vi "S4GUI.vi"(7 "Tab ObsEng":enum32{"Obs", "CCD modes", "Eng"}(tab)) -> ()   [LabVIEW 2018] (continued)
            n1128 = Equal?(x=w198, y=w197) -> (x = y?=w194:bool)
            n1129 = Or(x=w195, y=w194) -> (x .or. y?=w193:bool)
            n1130 = property on="Last Error" class="Str"(error in=w216, "Blinking"=w193) -> (error out=w199:errorcluster)  [unwired: 1 in, 1 out]
            n1131 = call "Read Instrument.lvclass.vi"("error in (no error)"=w199, "S4ACS_GUI in"=w201) -> ("error out"=w205:errorcluster, "Instrument.lvclass"=w204:refnum<class "Instrument.lvclass">, "S4ACS_GUI out"=w203:refnum<class "S4GUI.lvclass">)  [unwired: 7 in]
            n1132 = call-dynamic "Read mode.vi"("error in (no error)"=w205, "Instrument in"=w204) -> ("error out"=w202:errorcluster, "mode"=w206:bool)  [unwired: 7 in, 1 out]
            n1133 = while {
              tunnel: w206 -> [w249]
              shift-right: [w245] -> _
              shift-left: _ -> [w248]
              shift-right: [w246] -> _
              shift-left: _ -> [w247]
              stop <- TRUE stop-if-true
              n1134 = case shown="False" w249 {
                tunnel: w248 -> [w251 w270]
                tunnel: [w252 w269] -> w245
                tunnel: w247 -> [w254 w268]
                tunnel: [w253 w267] -> w246
                frame True {
                  # "polarimetria"
                  n1135 = case shown="False" w254 {
                    selector: w254 -> [w264 w266]
                    tunnel: [w263 w266] -> w253
                    tunnel: [FALSE FALSE] -> w252
                    tunnel: w251 -> [_ _]
                    frame False {
                      w261 = 11
                      w258 = 80
                      w257 = 12900
                      # "Valor médio\ndo curso do foco."
                      n1136 = local write "Start focus"(w257) -> ()
                      n1137 = local write "Step focus"(w258) -> ()
                      n1138 = local write "#steps"(w261) -> ()
                      n1139 = Quotient & Remainder(x=w261, y=2) -> (floor(x/y)=w259:i32)  [unwired: 1 out]
                      n1140 = Multiply(x=w258, y=w259) -> (x*y=w256:i32)
                      n1141 = Add(x=w257, y=w256) -> (x+y=w255:i32)
                      n1142 = local write "Target focus 2"(w255) -> ()
                      n1143 = local write "Target focus"(w255) -> ()
                      n1144 = Not(x=w264) -> (.not. x?=w263:bool)
                    }
                    frame True {
                    }
                  }
                }
                frame False {
                  # "fotometria"
                  n1145 = case shown="False" w270 {
                    selector: w270 -> [w279 w282]
                    tunnel: [w278 w282] -> w269
                    tunnel: w268 -> [_ _]
                    tunnel: [FALSE FALSE] -> w267
                    frame False {
                      w274 = 11
                      w273 = 100
                      w272 = 13400
                      # "Valor médio\ndo curso do foco."
                      n1146 = local write "Start focus"(w272) -> ()
                      n1147 = local write "Step focus"(w273) -> ()
                      n1148 = local write "#steps"(w274) -> ()
                      n1149 = Quotient & Remainder(x=w274, y=2) -> (floor(x/y)=w276:i32)  [unwired: 1 out]
                      n1150 = Multiply(x=w273, y=w276) -> (x*y=w275:i32)
                      n1151 = Add(x=w272, y=w275) -> (x+y=w271:i32)
                      n1152 = local write "Target focus"(w271) -> ()
                      n1153 = local write "Target focus 2"(w271) -> ()
                      n1154 = Not(x=w279) -> (.not. x?=w278:bool)
                    }
                    frame True {
                    }
                  }
                }
              }
            }
          }
        }
        n1155 = call-dynamic "Read exit.vi"("error in (no error)"=w141, "S4GUI in"=w142) -> ("error out"=w139:errorcluster, "exit"=w138:bool, "S4GUI out"=w140:refnum<class "S4GUI.lvclass">)  [unwired: 7 in]
      }
      event "Set CCD mode": Value Change {
        w1932 = i16 1 items=["Cooler OFF", "Cooler ON"] ("Cooler ON/OFF")
        w1946 = i16 1 items=["Cooler OFF", "Cooler ON"] ("Cooler ON/OFF")
        w1962 = i16 1 items=["Cooler OFF", "Cooler ON"] ("Cooler ON/OFF")
        w1982 = i16 1 items=["Cooler OFF", "Cooler ON"] ("Cooler ON/OFF")
        # "Sinaliza que houve requisição de SET CCD mode"
        n1156 = event-data() -> ()  [unwired: 1 in, 6 out]
        n1157 = call-dynamic "Write User Event.vi"("error in (no error)"=w2140, "User Event"="SET CCD mode ", "S4GUI in"=w2139) -> ("error out"=w1927:errorcluster, "S4GUI out"=w1926:refnum<class "S4GUI.lvclass">)  [unwired: 7 in]
        n1158 = call-dynamic "Write SET request.vi"("error in (no error)"=w1927, "SET request"=TRUE, "S4GUI in"=w1926) -> ("error out"=w1924:errorcluster, "S4GUI out"=w1925:refnum<class "S4GUI.lvclass">)  [unwired: 7 in]
        n1159 = call-dynamic "Read CCD mode.vi"("error in (no error)"=w1924, "S4GUI in"=w1925) -> ("error out"=w2137:errorcluster, "CCD mode"=w2138:T29, "S4GUI out"=w2136:refnum<class "S4GUI.lvclass">)  [unwired: 7 in]
        n1160 = Bundle By Name(cluster=w2138, "FTM"="FTM", "AQM"="AQM", "SZM"="SZM", "EM gain"="EM Gain") -> (w2135:T29)
        n1161 = call-dynamic "Write CCD mode.vi"("error in (no error)"=w2137, "CCD mode"=w2135, "S4GUI in"=w2136) -> ("error out"=w1993:errorcluster, "S4GUI out"=w1994:refnum<class "S4GUI.lvclass">)  [unwired: 7 in]
        n1162 = call-dynamic "LoadCCDmode.vi"("error in (no error)"=w1993, "S4GUI in"=w1994) -> ("error out"=w1992:errorcluster, "S4GUI out"=w1991:refnum<class "S4GUI.lvclass">)  [unwired: 8 in]
        n1163 = call-dynamic "Read Parameters CCD modes.vi"("error in (no error)"=w1992, "S4GUI in"=w1991) -> ("error out"=w1990:errorcluster, "Parameters CCD modes"=w1995:T5, "S4GUI out"=w1989:refnum<class "S4GUI.lvclass">)  [unwired: 7 in]
        n1164 = Unbundle By Name(w1995) -> ("CCD \nEM Mode"=w2127:u8, "Readout\nRate"=w1987:u8)
        n1165 = case shown="0, Default" w2127 {
          tunnel: [string[] ["30 MHz", "20 MHz", "10 MHz", "1 MHz"] ("Strings []") string[] ["1 MHz", "0.1 MHz"] ("Strings []")] -> w2128
          frame 0, Default {
          }
          frame 1 {
          }
        }
        n1166 = flat-sequence {
          tunnel: w2128 -> [w2274]
          tunnel: w2127 -> [w2275]
          tunnel: [w2275] -> w2129
          tunnel: w1995 -> [w2281]
          tunnel: [w2280] -> w1988
          tunnel: w2129 -> [w2278]
          tunnel: w1996 -> [w2279]
          tunnel: w1987 -> [w2276]
          frame #0 {
            n1167 = property on="Readout\nRate" class="Ring (strict)"("Strings []"=w2274) -> ()  [unwired: 2 in, 2 out]
            n1168 = property on="Readout\nRate" class="Ring (strict)"("Strings []"=w2274) -> ()  [unwired: 2 in, 2 out]
            n1169 = property on="Readout Rate 2" class="Ring (strict)"("Strings []"=w2274) -> ()  [unwired: 2 in, 2 out]
            n1170 = property on="Readout Rate" class="Ring (strict)"("Strings []"=w2274) -> ()  [unwired: 2 in, 2 out]
            n1171 = property on="Readout Rate 3" class="Ring (strict)"("Strings []"=w2274) -> ()  [unwired: 2 in, 2 out]
            n1172 = property on="Readout Rate 4" class="Ring (strict)"("Strings []"=w2274) -> ()  [unwired: 2 in, 2 out]
          }
          frame #1 {
            n1173 = Bundle By Name(cluster=w2281, "Readout\nRate"=w2276, "CCD \nEM Mode"=w2278) -> (w2280:T5)
            n1174 = disable-structure shown="Enabled" {
              disable-tunnel: w2279 -> [w2285 w2286]
              disable-tunnel: w2278 -> [w2284 _]
              disable-tunnel: [w2283 w2286] -> w2277
              disable-tunnel: w2276 -> [w2282 _]
              frame Disabled {
                n1175 = Bundle By Name(cluster=w2285, "Parameters.Readout\nRate"=w2282, "Parameters.CCD \nEM Mode"=w2284) -> (w2283:T8)
              }
              frame Enabled {
              }
            }
            n1176 = local write "Input Cluster"(w2277) -> ()
          }
        }
        n1177 = call-dynamic "Read InfoCCDmode.vi"("error in (no error)"=w1990, "S4GUI in"=w1989) -> ("error out"=w2130:errorcluster, "InfoCCDmode"=w1922:T2, "S4GUI out"=w2131:refnum<class "S4GUI.lvclass">)  [unwired: 7 in]
        "InfoCCDmode" <- w1922
        n1178 = Unbundle By Name(w1922) -> ("MinExpTime"=w1870:dbl)
        n1179 = call-dynamic "Read Parameters CCD modes.vi"("error in (no error)"=w2130, "S4GUI in"=w2131) -> ("error out"=w2124:errorcluster, "Parameters CCD modes"=→"Parameters CCD modes":T5, "S4GUI out"=w2125:refnum<class "S4GUI.lvclass">)  [unwired: 7 in]
        n1180 = local read "Input Cluster"() -> (w1996:T8)
        n1181 = call-dynamic "Write Parameters CCD modes.vi"("error in (no error)"=w2124, "Parameters CCD modes"=w1988, "S4GUI in"=w2125) -> ("error out"=w2103:errorcluster, "S4GUI out"=w2077:refnum<class "S4GUI.lvclass">)  [unwired: 7 in]
        n1182 = Unbundle By Name(w1988) -> ("Frame\nTransfer"=w2031:bool, "Pre-amplification\nGain"=w2030:u8, "Readout\nRate"=w2029:u8, "CCD \nEM Mode"=w2028:u8, "CCD\nEM Gain"=w2027:u16, "Image \nInitial Line"=w2026:u16, "Image\nInitial Column"=w2025:u16, "Image\nFinal Line"=w2014:u16, "Image\nFInal Column"=w2024:u16, "Vertical\nBinning"=w2023:u16, "Horizontal\nBinning"=w2022:u16)
        n1183 = call-dynamic "Read AcquisitionA.vi"("error in (no error)"=w2103, "S4ACS_GUI in"=w2077) -> ("error out"=w2012:errorcluster, "Acquisition.lvclass"=w2013:refnum<class "Acquisition.lvclass">, "S4ACS_GUI out"=w2123:refnum<class "S4GUI.lvclass">)  [unwired: 7 in]
        n1184 = call-dynamic "Read enabled.vi"("error in (no error)"=w2012, "Server in"=w2013) -> ("error out"=w2011:errorcluster, "enabled"=w2009:bool, "Server out"=w2010:refnum<class "Acquisition.lvclass">)  [unwired: 7 in]
        n1185 = call-dynamic "Read Channel.vi"("error in (no error)"=w2011, "Acquisition in"=w2010) -> ("error out"=w2120:errorcluster, "Channel.lvclass"=w2121:refnum<class "Channel.lvclass">, "Acquisition out"=w2122:refnum<class "Acquisition.lvclass">)  [unwired: 7 in]
        n1186 = call-dynamic "Read Interface.vi"("error in (no error)"=w2120, "Channel in"=w2121) -> ("error out"=w2106:errorcluster, "Interface.lvclass"=w2107:refnum<class "Interface.lvclass">, "Channel out"=w2101:refnum<class "Channel.lvclass">)  [unwired: 7 in]
        n1187 = call-dynamic "Write PREV_FT.vi"("error in (no error)"=w2106, "PREV_FT"=w2031, "Interface in"=w2107) -> ("error out"=w1985:errorcluster, "Interface out"=w1984:refnum<class "Interface.lvclass">)  [unwired: 7 in]
        n1188 = call-dynamic "Write Cooler ON_OFF.vi"("error in (no error)"=w1985, "Cooler ON/OFF"=w1982, "Interface in"=w1984) -> ("error out"=w1983:errorcluster, "Interface out"=w1981:refnum<class "Interface.lvclass">)  [unwired: 7 in]
        n1189 = call-dynamic "Read target cluster.vi"("error in (no error)"=w1983, "Channel in"=w2101) -> ("error out"=w2099:errorcluster, "target cluster"=w2098:T30, "Channel out"=w2100:refnum<class "Channel.lvclass">)  [unwired: 7 in]
        n1190 = Bundle By Name(cluster=w2098, "FRAME_TRANSFER"=w2031, "PREAMP"=w2030, "READOUT_RATE"=w2029, "EM_MODE"=w2028, "EM_GAIN"=w2027, "INITIAL_LINE"=w2026, "INITIAL_COLUMN"=w2025, "FINAL_LINE"=w2014, "FINAL_COLUMN"=w2024, "VBIN"=w2023, "HBIN"=w2022) -> (w1978:T30)
        n1191 = call-dynamic "Write target cluster.vi"("error in (no error)"=w2099, "target cluster"=w1978, "Channel in"=w2100) -> ("error out"=w1979:errorcluster, "Channel out"=w2105:refnum<class "Channel.lvclass">)  [unwired: 7 in]
        n1192 = call-dynamic "Set CCD_Config.vi"("error in (no error)"=w1979, "input cluster"=w1978, "Interface in"=w1981) -> ("error out"=w1968:errorcluster, "Interface out"=w1980:refnum<class "Interface.lvclass">)  [unwired: 7 in]
        n1193 = Flatten To String(anything=w1978, error in (no error)=w1979) -> (data string=w2115:string)  [unwired: 2 in, 2 out]
        n1194 = call "Write flatted cluster.vi"("error in (no error)"=w1968, "flatted cluster"=w2115, "Interface in"=w1980) -> ("error out"=w1917:errorcluster, "Interface out"=w1918:refnum<class "Interface.lvclass">)  [unwired: 7 in]
        n1195 = call "Read Exposure Time.vi"("error in (no error)"=w1917, "Interface in"=w1918) -> ("error out"=w1915:errorcluster, "Exposure Time"=w1920:dbl, "Interface out"=w1916:refnum<class "Interface.lvclass">)  [unwired: 7 in]
        n1196 = Greater Or Equal?(x=w1920, y=w1870) -> (x >= y?=w1921:bool)
        n1197 = Select(t=w1920, s=w1921, f=w1870) -> (s? t:f=w1919:dbl)
        n1198 = local write "Exptime ch1"(w1919) -> ()
        n1199 = call "Write Exposure Time.vi"("error in (no error)"=w1915, "Exposure Time"=w1919, "Interface in"=w1916) -> ("error out"=w1914:errorcluster, "Interface out"=w1913:refnum<class "Interface.lvclass">)  [unwired: 7 in]
        n1200 = call-dynamic "Write Interface.vi"("error in (no error)"=w1914, "Interface.lvclass"=w1913, "Channel in"=w2105) -> ("error out"=w2111:errorcluster, "Channel out"=w2113:refnum<class "Channel.lvclass">)  [unwired: 7 in]
        n1201 = call "Write section_name.vi"("error in (no error)"=w2111, "section_name"="CCD_ACS1", "Channel in"=w2113) -> ("error out"=w2110:errorcluster, "Channel out"=w2112:refnum<class "Channel.lvclass">)  [unwired: 7 in]
        n1202 = call-dynamic "save config.vi"("error in (no error)"=w2110, "file config"="lastsaved.cfg", "Channel in"=w2112) -> ("error out"=w1976:errorcluster, "Channel out"=w1977:refnum<class "Channel.lvclass">)  [unwired: 7 in]
        n1203 = call-dynamic "ValidateConfig.vi"("error in (no error)"=w1976, "Channel in"=w1977) -> ("error out"=w1974:errorcluster, "Channel out"=w1975:refnum<class "Channel.lvclass">)  [unwired: 7 in, 1 out]
        n1204 = call-dynamic "Save Temp.vi"("error in (no error)"=w1974, "temp file"="lasttemp.cfg" ("file config"), "Channel in"=w1975) -> ("error out"=w1973:errorcluster, "Channel out"=w1972:refnum<class "Channel.lvclass">)  [unwired: 7 in]
        n1205 = case shown="True" w2009 {
          tunnel: [w2242 w2267] -> w2119
          tunnel: [w2241 w2266] -> w2118
          tunnel: w1972 -> [w2242 w2265]
          tunnel: w1973 -> [w2241 w2264]
          frame False {
          }
          frame True {
            # "Esvazia\na fila."
            n1206 = call-dynamic "Read State Machine.vi"("error in (no error)"=w2264, "Device in"=w2265) -> ("error out"=w2258:errorcluster, "State Machine.lvclass"=w2261:refnum<class "State Machine.lvclass">, "Device out"=w2271:refnum<class "Channel.lvclass">)  [unwired: 7 in]
            n1207 = call-dynamic "Read ref StatesQueue.vi"("error in (no error)"=w2258, "State Machine in"=w2261) -> ("error out"=w2249:errorcluster, "ref StatesQueue"=w2251:refnum<queue>, "State Machine out"=w2260:refnum<class "State Machine.lvclass">)  [unwired: 7 in]
            n1208 = Flush Queue(queue=w2251, error in (no error)=w2249) -> (queue out=w2250:refnum<queue>, error out=w2248:errorcluster)  [unwired: 1 out]
            n1209 = Enqueue Element(queue=w2250, element=u32 60 ("State"), error in (no error)=w2248) -> (queue out=w2263:refnum<queue>, error out=w2257:errorcluster)  [unwired: 1 in, 1 out]
            n1210 = Enqueue Element(queue=w2263, element=u32 45 ("State"), error in (no error)=w2257) -> (queue out=w2262:refnum<queue>, error out=w2256:errorcluster)  [unwired: 1 in, 1 out]
            n1211 = Enqueue Element(queue=w2262, element=u32 35 ("State"), error in (no error)=w2256) -> (queue out=w2246:refnum<queue>, error out=w2245:errorcluster)  [unwired: 1 in, 1 out]
            n1212 = Enqueue Element(queue=w2246, element=u32 37 ("State"), error in (no error)=w2245) -> (queue out=w2243:refnum<queue>, error out=w2244:errorcluster)  [unwired: 1 in, 1 out]
            n1213 = call-dynamic "Write ref StatesQueue.vi"("error in (no error)"=w2244, "ref StatesQueue"=w2243, "State Machine in"=w2260) -> ("error out"=w2252:errorcluster, "State Machine out"=w2259:refnum<class "State Machine.lvclass">)  [unwired: 7 in]
            n1214 = disable-structure shown="Enabled" {
              disable-tunnel: [0 ("State") 45] -> w2268
              frame Enabled {
                # "Vai pra 0 para que\nos estados da fila \nsejam retirados."
              }
              frame Disabled {
                # "Verifica Texp\nantes de tudo."
              }
            }
            n1215 = call-dynamic "Write State.vi"("error in (no error)"=w2252, "State"=w2268, "State Machine in"=w2259) -> ("error out"=w2269:errorcluster, "State Machine out"=w2270:refnum<class "State Machine.lvclass">)  [unwired: 7 in]
            n1216 = call-dynamic "Write State Machine.vi"("error in (no error)"=w2269, "State Machine.lvclass"=w2270, "Device in"=w2271) -> ("error out"=w2266:errorcluster, "Device out"=w2267:refnum<class "Channel.lvclass">)  [unwired: 7 in]
          }
        }
        n1217 = call-dynamic "Write Channel.vi"("error in (no error)"=w2118, "Channel.lvclass"=w2119, "Acquisition in"=w2122) -> ("error out"=w2117:errorcluster, "Acquisition out"=w2116:refnum<class "Acquisition.lvclass">)  [unwired: 7 in]
        n1218 = call-dynamic "Write AcquisitionA.vi"("error in (no error)"=w2117, "Acquisition.lvclass"=w2116, "S4ACS_GUI in"=w2123) -> ("error out"=w2019:errorcluster, "S4ACS_GUI out"=w2076:refnum<class "S4GUI.lvclass">)  [unwired: 7 in]
        n1219 = call "Read AcquisitionB.vi"("error in (no error)"=errorcluster {"status"=FALSE, "code"=0, "source"=""}, "S4ACS_GUI in"=w2076) -> ("error out"=w2005:errorcluster, "Acquisition.lvclass"=w2008:refnum<class "Acquisition.lvclass">, "S4ACS_GUI out"=w2097:refnum<class "S4GUI.lvclass">)  [unwired: 7 in]
        n1220 = call-dynamic "Read enabled.vi"("error in (no error)"=w2005, "Server in"=w2008) -> ("error out"=w2006:errorcluster, "enabled"=w1898:bool, "Server out"=w2007:refnum<class "Acquisition.lvclass">)  [unwired: 7 in]
        n1221 = call-dynamic "Read Channel.vi"("error in (no error)"=w2006, "Acquisition in"=w2007) -> ("error out"=w2094:errorcluster, "Channel.lvclass"=w2095:refnum<class "Channel.lvclass">, "Acquisition out"=w2096:refnum<class "Acquisition.lvclass">)  [unwired: 7 in]
        n1222 = call-dynamic "Read Interface.vi"("error in (no error)"=w2094, "Channel in"=w2095) -> ("error out"=w2083:errorcluster, "Interface.lvclass"=w2084:refnum<class "Interface.lvclass">, "Channel out"=w2081:refnum<class "Channel.lvclass">)  [unwired: 7 in]
        n1223 = call-dynamic "Write PREV_FT.vi"("error in (no error)"=w2083, "PREV_FT"=w2031, "Interface in"=w2084) -> ("error out"=w1963:errorcluster, "Interface out"=w1965:refnum<class "Interface.lvclass">)  [unwired: 7 in]
        n1224 = call-dynamic "Write Cooler ON_OFF.vi"("error in (no error)"=w1963, "Cooler ON/OFF"=w1962, "Interface in"=w1965) -> ("error out"=w1961:errorcluster, "Interface out"=w1964:refnum<class "Interface.lvclass">)  [unwired: 7 in]
        n1225 = call-dynamic "Read target cluster.vi"("error in (no error)"=w1961, "Channel in"=w2081) -> ("error out"=w2079:errorcluster, "target cluster"=w2078:T30, "Channel out"=w2080:refnum<class "Channel.lvclass">)  [unwired: 7 in]
        n1226 = Bundle By Name(cluster=w2078, "FRAME_TRANSFER"=w2031, "PREAMP"=w2030, "READOUT_RATE"=w2029, "EM_MODE"=w2028, "EM_GAIN"=w2027, "INITIAL_LINE"=w2026, "INITIAL_COLUMN"=w2025, "FINAL_LINE"=w2014, "FINAL_COLUMN"=w2024, "VBIN"=w2023, "HBIN"=w2022) -> (w1966:T30)
        n1227 = call-dynamic "Write target cluster.vi"("error in (no error)"=w2079, "target cluster"=w1966, "Channel in"=w2080) -> ("error out"=w1969:errorcluster, "Channel out"=w2082:refnum<class "Channel.lvclass">)  [unwired: 7 in]
        n1228 = call-dynamic "Set CCD_Config.vi"("error in (no error)"=w1969, "input cluster"=w1966, "Interface in"=w1964) -> ("error out"=w1967:errorcluster, "Interface out"=w1970:refnum<class "Interface.lvclass">)  [unwired: 7 in]
        n1229 = Flatten To String(anything=w1966, error in (no error)=w1969) -> (data string=w2091:string)  [unwired: 2 in, 2 out]
        n1230 = call "Write flatted cluster.vi"("error in (no error)"=w1967, "flatted cluster"=w2091, "Interface in"=w1970) -> ("error out"=w1891:errorcluster, "Interface out"=w1892:refnum<class "Interface.lvclass">)  [unwired: 7 in]
        n1231 = call "Read Exposure Time.vi"("error in (no error)"=w1891, "Interface in"=w1892) -> ("error out"=w1912:errorcluster, "Exposure Time"=w1893:dbl, "Interface out"=w1911:refnum<class "Interface.lvclass">)  [unwired: 7 in]
        n1232 = Greater Or Equal?(x=w1893, y=w1870) -> (x >= y?=w1909:bool)
        n1233 = Select(t=w1893, s=w1909, f=w1870) -> (s? t:f=w1910:dbl)
        n1234 = local write "Exptime ch2"(w1910) -> ()
        n1235 = call "Write Exposure Time.vi"("error in (no error)"=w1912, "Exposure Time"=w1910, "Interface in"=w1911) -> ("error out"=w1890:errorcluster, "Interface out"=w1889:refnum<class "Interface.lvclass">)  [unwired: 7 in]
        n1236 = call-dynamic "Write Interface.vi"("error in (no error)"=w1890, "Interface.lvclass"=w1889, "Channel in"=w2082) -> ("error out"=w2087:errorcluster, "Channel out"=w2089:refnum<class "Channel.lvclass">)  [unwired: 7 in]
        n1237 = call "Write section_name.vi"("error in (no error)"=w2087, "section_name"="CCD_ACS2", "Channel in"=w2089) -> ("error out"=w2086:errorcluster, "Channel out"=w2088:refnum<class "Channel.lvclass">)  [unwired: 7 in]
        n1238 = call-dynamic "save config.vi"("error in (no error)"=w2086, "file config"="lastsaved.cfg", "Channel in"=w2088) -> ("error out"=w1956:errorcluster, "Channel out"=w1957:refnum<class "Channel.lvclass">)  [unwired: 7 in]
        n1239 = call-dynamic "ValidateConfig.vi"("error in (no error)"=w1956, "Channel in"=w1957) -> ("error out"=w1959:errorcluster, "Channel out"=w1960:refnum<class "Channel.lvclass">)  [unwired: 7 in, 1 out]
        n1240 = call-dynamic "Save Temp.vi"("error in (no error)"=w1959, "temp file"="lasttemp.cfg" ("file config"), "Channel in"=w1960) -> ("error out"=w1896:errorcluster, "Channel out"=w1897:refnum<class "Channel.lvclass">)  [unwired: 7 in]
        n1241 = case shown="True" w1898 {
          tunnel: [w2176 w2201] -> w1895
          tunnel: [w2175 w2200] -> w1894
          tunnel: w1897 -> [w2176 w2199]
          tunnel: w1896 -> [w2175 w2198]
          frame False {
          }
          frame True {
            # "Esvazia\na fila."
            n1242 = call-dynamic "Read State Machine.vi"("error in (no error)"=w2198, "Device in"=w2199) -> ("error out"=w2192:errorcluster, "State Machine.lvclass"=w2195:refnum<class "State Machine.lvclass">, "Device out"=w2205:refnum<class "Channel.lvclass">)  [unwired: 7 in]
            n1243 = call-dynamic "Read ref StatesQueue.vi"("error in (no error)"=w2192, "State Machine in"=w2195) -> ("error out"=w2182:errorcluster, "ref StatesQueue"=w2184:refnum<queue>, "State Machine out"=w2194:refnum<class "State Machine.lvclass">)  [unwired: 7 in]
            n1244 = Flush Queue(queue=w2184, error in (no error)=w2182) -> (queue out=w2183:refnum<queue>, error out=w2181:errorcluster)  [unwired: 1 out]
            n1245 = Enqueue Element(queue=w2183, element=u32 60 ("State"), error in (no error)=w2181) -> (queue out=w2197:refnum<queue>, error out=w2191:errorcluster)  [unwired: 1 in, 1 out]
            n1246 = Enqueue Element(queue=w2197, element=u32 45 ("State"), error in (no error)=w2191) -> (queue out=w2196:refnum<queue>, error out=w2190:errorcluster)  [unwired: 1 in, 1 out]
            n1247 = Enqueue Element(queue=w2196, element=u32 35 ("State"), error in (no error)=w2190) -> (queue out=w2189:refnum<queue>, error out=w2179:errorcluster)  [unwired: 1 in, 1 out]
            n1248 = Enqueue Element(queue=w2189, element=u32 37, error in (no error)=w2179) -> (queue out=w2180:refnum<queue>, error out=w2178:errorcluster)  [unwired: 1 in, 1 out]
            n1249 = call-dynamic "Write ref StatesQueue.vi"("error in (no error)"=w2178, "ref StatesQueue"=w2180, "State Machine in"=w2194) -> ("error out"=w2185:errorcluster, "State Machine out"=w2193:refnum<class "State Machine.lvclass">)  [unwired: 7 in]
            n1250 = disable-structure shown="Enabled" {
              disable-tunnel: [0 ("State") 45] -> w2202
              frame Enabled {
                # "Vai pra 0 para que\nos estados da fila \nsejam retirados."
              }
              frame Disabled {
                # "Verifica Texp\nantes de tudo."
              }
            }
            n1251 = call-dynamic "Write State.vi"("error in (no error)"=w2185, "State"=w2202, "State Machine in"=w2193) -> ("error out"=w2203:errorcluster, "State Machine out"=w2204:refnum<class "State Machine.lvclass">)  [unwired: 7 in]
            n1252 = call-dynamic "Write State Machine.vi"("error in (no error)"=w2203, "State Machine.lvclass"=w2204, "Device in"=w2205) -> ("error out"=w2200:errorcluster, "Device out"=w2201:refnum<class "Channel.lvclass">)  [unwired: 7 in]
          }
        }
        n1253 = call-dynamic "Write Channel.vi"("error in (no error)"=w1894, "Channel.lvclass"=w1895, "Acquisition in"=w2096) -> ("error out"=w2093:errorcluster, "Acquisition out"=w2092:refnum<class "Acquisition.lvclass">)  [unwired: 7 in]
        n1254 = call "Write AcquisitionB.vi"("error in (no error)"=w2093, "Acquisition.lvclass"=w2092, "S4ACS_GUI in"=w2097) -> ("error out"=w2018:errorcluster, "S4ACS_GUI out"=w2053:refnum<class "S4GUI.lvclass">)  [unwired: 7 in]
        n1255 = call-dynamic "Read AcquisitionC.vi"("error in (no error)"=errorcluster {"status"=FALSE, "code"=0, "source"=""}, "S4ACS_GUI in"=w2053) -> ("error out"=w2002:errorcluster, "Acquisition.lvclass"=w2004:refnum<class "Acquisition.lvclass">, "S4ACS_GUI out"=w2074:refnum<class "S4GUI.lvclass">)  [unwired: 7 in]
        n1256 = call-dynamic "Read enabled.vi"("error in (no error)"=w2002, "Server in"=w2004) -> ("error out"=w2001:errorcluster, "enabled"=w1888:bool, "Server out"=w2003:refnum<class "Acquisition.lvclass">)  [unwired: 7 in]
        n1257 = call-dynamic "Read Channel.vi"("error in (no error)"=w2001, "Acquisition in"=w2003) -> ("error out"=w2071:errorcluster, "Channel.lvclass"=w2072:refnum<class "Channel.lvclass">, "Acquisition out"=w2073:refnum<class "Acquisition.lvclass">)  [unwired: 7 in]
        n1258 = call-dynamic "Read Interface.vi"("error in (no error)"=w2071, "Channel in"=w2072) -> ("error out"=w2060:errorcluster, "Interface.lvclass"=w2061:refnum<class "Interface.lvclass">, "Channel out"=w2058:refnum<class "Channel.lvclass">)  [unwired: 7 in]
        n1259 = call-dynamic "Write PREV_FT.vi"("error in (no error)"=w2060, "PREV_FT"=w2031, "Interface in"=w2061) -> ("error out"=w1943:errorcluster, "Interface out"=w1945:refnum<class "Interface.lvclass">)  [unwired: 7 in]
        n1260 = call-dynamic "Write Cooler ON_OFF.vi"("error in (no error)"=w1943, "Cooler ON/OFF"=w1946, "Interface in"=w1945) -> ("error out"=w1942:errorcluster, "Interface out"=w1944:refnum<class "Interface.lvclass">)  [unwired: 7 in]
        n1261 = call-dynamic "Read target cluster.vi"("error in (no error)"=w1942, "Channel in"=w2058) -> ("error out"=w2056:errorcluster, "target cluster"=w2055:T30, "Channel out"=w2057:refnum<class "Channel.lvclass">)  [unwired: 7 in]
        n1262 = Bundle By Name(cluster=w2055, "FRAME_TRANSFER"=w2031, "PREAMP"=w2030, "READOUT_RATE"=w2029, "EM_MODE"=w2028, "EM_GAIN"=w2027, "INITIAL_LINE"=w2026, "INITIAL_COLUMN"=w2025, "FINAL_LINE"=w2014, "FINAL_COLUMN"=w2024, "VBIN"=w2023, "HBIN"=w2022) -> (w1950:T30)
        n1263 = call-dynamic "Write target cluster.vi"("error in (no error)"=w2056, "target cluster"=w1950, "Channel in"=w2057) -> ("error out"=w1949:errorcluster, "Channel out"=w2059:refnum<class "Channel.lvclass">)  [unwired: 7 in]
        n1264 = call-dynamic "Set CCD_Config.vi"("error in (no error)"=w1949, "input cluster"=w1950, "Interface in"=w1944) -> ("error out"=w1948:errorcluster, "Interface out"=w1947:refnum<class "Interface.lvclass">)  [unwired: 7 in]
        n1265 = Flatten To String(anything=w1950, error in (no error)=w1949) -> (data string=w2068:string)  [unwired: 2 in, 2 out]
        n1266 = call "Write flatted cluster.vi"("error in (no error)"=w1948, "flatted cluster"=w2068, "Interface in"=w1947) -> ("error out"=w1882:errorcluster, "Interface out"=w1883:refnum<class "Interface.lvclass">)  [unwired: 7 in]
        n1267 = call "Read Exposure Time.vi"("error in (no error)"=w1882, "Interface in"=w1883) -> ("error out"=w1904:errorcluster, "Exposure Time"=w1907:dbl, "Interface out"=w1905:refnum<class "Interface.lvclass">)  [unwired: 7 in]
        n1268 = Greater Or Equal?(x=w1907, y=w1870) -> (x >= y?=w1908:bool)
        n1269 = Select(t=w1907, s=w1908, f=w1870) -> (s? t:f=w1906:dbl)
        n1270 = local write "Exptime ch3"(w1906) -> ()
        n1271 = call "Write Exposure Time.vi"("error in (no error)"=w1904, "Exposure Time"=w1906, "Interface in"=w1905) -> ("error out"=w1880:errorcluster, "Interface out"=w1881:refnum<class "Interface.lvclass">)  [unwired: 7 in]
        n1272 = call-dynamic "Write Interface.vi"("error in (no error)"=w1880, "Interface.lvclass"=w1881, "Channel in"=w2059) -> ("error out"=w2064:errorcluster, "Channel out"=w2066:refnum<class "Channel.lvclass">)  [unwired: 7 in]
        n1273 = call "Write section_name.vi"("error in (no error)"=w2064, "section_name"="CCD_ACS3", "Channel in"=w2066) -> ("error out"=w2063:errorcluster, "Channel out"=w2065:refnum<class "Channel.lvclass">)  [unwired: 7 in]
        n1274 = call-dynamic "save config.vi"("error in (no error)"=w2063, "file config"="lastsaved.cfg", "Channel in"=w2065) -> ("error out"=w1951:errorcluster, "Channel out"=w1952:refnum<class "Channel.lvclass">)  [unwired: 7 in]
        n1275 = call-dynamic "ValidateConfig.vi"("error in (no error)"=w1951, "Channel in"=w1952) -> ("error out"=w1954:errorcluster, "Channel out"=w1955:refnum<class "Channel.lvclass">)  [unwired: 7 in, 1 out]
        n1276 = call-dynamic "Save Temp.vi"("error in (no error)"=w1954, "temp file"="lasttemp.cfg" ("file config"), "Channel in"=w1955) -> ("error out"=w1886:errorcluster, "Channel out"=w1887:refnum<class "Channel.lvclass">)  [unwired: 7 in]
        n1277 = case shown="True" w1888 {
          tunnel: [w2143 w2168] -> w1885
          tunnel: [w2142 w2167] -> w1884
          tunnel: w1887 -> [w2143 w2166]
          tunnel: w1886 -> [w2142 w2165]
          frame False {
          }
          frame True {
            # "Esvazia\na fila."
            n1278 = call-dynamic "Read State Machine.vi"("error in (no error)"=w2165, "Device in"=w2166) -> ("error out"=w2159:errorcluster, "State Machine.lvclass"=w2162:refnum<class "State Machine.lvclass">, "Device out"=w2172:refnum<class "Channel.lvclass">)  [unwired: 7 in]
            n1279 = call-dynamic "Read ref StatesQueue.vi"("error in (no error)"=w2159, "State Machine in"=w2162) -> ("error out"=w2149:errorcluster, "ref StatesQueue"=w2151:refnum<queue>, "State Machine out"=w2161:refnum<class "State Machine.lvclass">)  [unwired: 7 in]
            n1280 = Flush Queue(queue=w2151, error in (no error)=w2149) -> (queue out=w2150:refnum<queue>, error out=w2148:errorcluster)  [unwired: 1 out]
            n1281 = Enqueue Element(queue=w2150, element=u32 60 ("State"), error in (no error)=w2148) -> (queue out=w2164:refnum<queue>, error out=w2158:errorcluster)  [unwired: 1 in, 1 out]
            n1282 = Enqueue Element(queue=w2164, element=u32 45 ("State"), error in (no error)=w2158) -> (queue out=w2163:refnum<queue>, error out=w2157:errorcluster)  [unwired: 1 in, 1 out]
            n1283 = Enqueue Element(queue=w2163, element=u32 35 ("State"), error in (no error)=w2157) -> (queue out=w2156:refnum<queue>, error out=w2146:errorcluster)  [unwired: 1 in, 1 out]
            n1284 = Enqueue Element(queue=w2156, element=u32 37, error in (no error)=w2146) -> (queue out=w2147:refnum<queue>, error out=w2145:errorcluster)  [unwired: 1 in, 1 out]
            n1285 = call-dynamic "Write ref StatesQueue.vi"("error in (no error)"=w2145, "ref StatesQueue"=w2147, "State Machine in"=w2161) -> ("error out"=w2152:errorcluster, "State Machine out"=w2160:refnum<class "State Machine.lvclass">)  [unwired: 7 in]
            n1286 = disable-structure shown="Enabled" {
              disable-tunnel: [0 ("State") 45] -> w2169
              frame Enabled {
                # "Vai pra 0 para que\nos estados da fila \nsejam retirados."
              }
              frame Disabled {
                # "Verifica Texp\nantes de tudo."
              }
            }
            n1287 = call-dynamic "Write State.vi"("error in (no error)"=w2152, "State"=w2169, "State Machine in"=w2160) -> ("error out"=w2170:errorcluster, "State Machine out"=w2171:refnum<class "State Machine.lvclass">)  [unwired: 7 in]
            n1288 = call-dynamic "Write State Machine.vi"("error in (no error)"=w2170, "State Machine.lvclass"=w2171, "Device in"=w2172) -> ("error out"=w2167:errorcluster, "Device out"=w2168:refnum<class "Channel.lvclass">)  [unwired: 7 in]
          }
        }
        n1289 = call-dynamic "Write Channel.vi"("error in (no error)"=w1884, "Channel.lvclass"=w1885, "Acquisition in"=w2073) -> ("error out"=w2070:errorcluster, "Acquisition out"=w2069:refnum<class "Acquisition.lvclass">)  [unwired: 7 in]
        n1290 = call-dynamic "Write AcquisitionC.vi"("error in (no error)"=w2070, "Acquisition.lvclass"=w2069, "S4ACS_GUI in"=w2074) -> ("error out"=w2017:errorcluster, "S4ACS_GUI out"=w2021:refnum<class "S4GUI.lvclass">)  [unwired: 7 in]
        n1291 = call-dynamic "Read AcquisitionD.vi"("error in (no error)"=errorcluster {"status"=FALSE, "code"=0, "source"=""}, "S4ACS_GUI in"=w2021) -> ("error out"=w1998:errorcluster, "Acquisition.lvclass"=w2000:refnum<class "Acquisition.lvclass">, "S4ACS_GUI out"=w2052:refnum<class "S4GUI.lvclass">)  [unwired: 7 in]
        n1292 = call-dynamic "Read enabled.vi"("error in (no error)"=w1998, "Server in"=w2000) -> ("error out"=w1997:errorcluster, "enabled"=w1879:bool, "Server out"=w1999:refnum<class "Acquisition.lvclass">)  [unwired: 7 in]
        n1293 = call-dynamic "Read Channel.vi"("error in (no error)"=w1997, "Acquisition in"=w1999) -> ("error out"=w2049:errorcluster, "Channel.lvclass"=w2050:refnum<class "Channel.lvclass">, "Acquisition out"=w2051:refnum<class "Acquisition.lvclass">)  [unwired: 7 in]
        n1294 = call-dynamic "Read Interface.vi"("error in (no error)"=w2049, "Channel in"=w2050) -> ("error out"=w2038:errorcluster, "Interface.lvclass"=w2039:refnum<class "Interface.lvclass">, "Channel out"=w2036:refnum<class "Channel.lvclass">)  [unwired: 7 in]
        n1295 = call-dynamic "Write PREV_FT.vi"("error in (no error)"=w2038, "PREV_FT"=w2031, "Interface in"=w2039) -> ("error out"=w1931:errorcluster, "Interface out"=w1930:refnum<class "Interface.lvclass">)  [unwired: 7 in]
        n1296 = call-dynamic "Write Cooler ON_OFF.vi"("error in (no error)"=w1931, "Cooler ON/OFF"=w1932, "Interface in"=w1930) -> ("error out"=w1928:errorcluster, "Interface out"=w1929:refnum<class "Interface.lvclass">)  [unwired: 7 in]
        n1297 = call-dynamic "Read target cluster.vi"("error in (no error)"=w1928, "Channel in"=w2036) -> ("error out"=w2034:errorcluster, "target cluster"=w2033:T30, "Channel out"=w2035:refnum<class "Channel.lvclass">)  [unwired: 7 in]
        n1298 = Bundle By Name(cluster=w2033, "FRAME_TRANSFER"=w2031, "PREAMP"=w2030, "READOUT_RATE"=w2029, "EM_MODE"=w2028, "EM_GAIN"=w2027, "INITIAL_LINE"=w2026, "INITIAL_COLUMN"=w2025, "FINAL_LINE"=w2014, "FINAL_COLUMN"=w2024, "VBIN"=w2023, "HBIN"=w2022) -> (w1933:T30)
        n1299 = call-dynamic "Write target cluster.vi"("error in (no error)"=w2034, "target cluster"=w1933, "Channel in"=w2035) -> ("error out"=w1934:errorcluster, "Channel out"=w2037:refnum<class "Channel.lvclass">)  [unwired: 7 in]
        n1300 = call-dynamic "Set CCD_Config.vi"("error in (no error)"=w1934, "input cluster"=w1933, "Interface in"=w1929) -> ("error out"=w1935:errorcluster, "Interface out"=w1936:refnum<class "Interface.lvclass">)  [unwired: 7 in]
        n1301 = Flatten To String(anything=w1933, error in (no error)=w1934) -> (data string=w2046:string)  [unwired: 2 in, 2 out]
        n1302 = call "Write flatted cluster.vi"("error in (no error)"=w1935, "flatted cluster"=w2046, "Interface in"=w1936) -> ("error out"=w1873:errorcluster, "Interface out"=w1874:refnum<class "Interface.lvclass">)  [unwired: 7 in]
        n1303 = call "Read Exposure Time.vi"("error in (no error)"=w1873, "Interface in"=w1874) -> ("error out"=w1903:errorcluster, "Exposure Time"=w1900:dbl, "Interface out"=w1902:refnum<class "Interface.lvclass">)  [unwired: 7 in]
        n1304 = Greater Or Equal?(x=w1900, y=w1870) -> (x >= y?=w1899:bool)
        n1305 = Select(t=w1900, s=w1899, f=w1870) -> (s? t:f=w1901:dbl)
        n1306 = local write "Exptime ch4"(w1901) -> ()
        n1307 = call "Write Exposure Time.vi"("error in (no error)"=w1903, "Exposure Time"=w1901, "Interface in"=w1902) -> ("error out"=w1871:errorcluster, "Interface out"=w1872:refnum<class "Interface.lvclass">)  [unwired: 7 in]
        n1308 = call-dynamic "Write Interface.vi"("error in (no error)"=w1871, "Interface.lvclass"=w1872, "Channel in"=w2037) -> ("error out"=w2042:errorcluster, "Channel out"=w2044:refnum<class "Channel.lvclass">)  [unwired: 7 in]
        n1309 = call "Write section_name.vi"("error in (no error)"=w2042, "section_name"="CCD_ACS4", "Channel in"=w2044) -> ("error out"=w2041:errorcluster, "Channel out"=w2043:refnum<class "Channel.lvclass">)  [unwired: 7 in]
        n1310 = call-dynamic "save config.vi"("error in (no error)"=w2041, "file config"="lastsaved.cfg", "Channel in"=w2043) -> ("error out"=w1937:errorcluster, "Channel out"=w1938:refnum<class "Channel.lvclass">)  [unwired: 7 in]
        n1311 = call-dynamic "ValidateConfig.vi"("error in (no error)"=w1937, "Channel in"=w1938) -> ("error out"=w1940:errorcluster, "Channel out"=w1941:refnum<class "Channel.lvclass">)  [unwired: 7 in, 1 out]
        n1312 = call-dynamic "Save Temp.vi"("error in (no error)"=w1940, "temp file"="lasttemp.cfg" ("file config"), "Channel in"=w1941) -> ("error out"=w1876:errorcluster, "Channel out"=w1875:refnum<class "Channel.lvclass">)  [unwired: 7 in]
        n1313 = case shown="True" w1879 {
          tunnel: [w2208 w2234] -> w1878
          tunnel: [w2209 w2233] -> w1877
          tunnel: w1876 -> [w2209 w2232]
          tunnel: w1875 -> [w2208 w2214]
          frame False {
          }
          frame True {
            # "Esvazia\na fila."
            n1314 = call-dynamic "Read State Machine.vi"("error in (no error)"=w2232, "Device in"=w2214) -> ("error out"=w2226:errorcluster, "State Machine.lvclass"=w2229:refnum<class "State Machine.lvclass">, "Device out"=w2238:refnum<class "Channel.lvclass">)  [unwired: 7 in]
            n1315 = call-dynamic "Read ref StatesQueue.vi"("error in (no error)"=w2226, "State Machine in"=w2229) -> ("error out"=w2216:errorcluster, "ref StatesQueue"=w2218:refnum<queue>, "State Machine out"=w2228:refnum<class "State Machine.lvclass">)  [unwired: 7 in]
            n1316 = Flush Queue(queue=w2218, error in (no error)=w2216) -> (queue out=w2217:refnum<queue>, error out=w2215:errorcluster)  [unwired: 1 out]
            n1317 = Enqueue Element(queue=w2217, element=u32 60 ("State"), error in (no error)=w2215) -> (queue out=w2231:refnum<queue>, error out=w2225:errorcluster)  [unwired: 1 in, 1 out]
            n1318 = Enqueue Element(queue=w2231, element=u32 45 ("State"), error in (no error)=w2225) -> (queue out=w2230:refnum<queue>, error out=w2224:errorcluster)  [unwired: 1 in, 1 out]
            n1319 = Enqueue Element(queue=w2230, element=u32 35 ("State"), error in (no error)=w2224) -> (queue out=w2223:refnum<queue>, error out=w2212:errorcluster)  [unwired: 1 in, 1 out]
            n1320 = Enqueue Element(queue=w2223, element=u32 37, error in (no error)=w2212) -> (queue out=w2213:refnum<queue>, error out=w2211:errorcluster)  [unwired: 1 in, 1 out]
            n1321 = call-dynamic "Write ref StatesQueue.vi"("error in (no error)"=w2211, "ref StatesQueue"=w2213, "State Machine in"=w2228) -> ("error out"=w2219:errorcluster, "State Machine out"=w2227:refnum<class "State Machine.lvclass">)  [unwired: 7 in]
            n1322 = disable-structure shown="Enabled" {
              disable-tunnel: [0 ("State") 45] -> w2235
              frame Enabled {
                # "Vai pra 0 para que\nos estados da fila \nsejam retirados."
              }
              frame Disabled {
                # "Verifica Texp\nantes de tudo."
              }
            }
            n1323 = call-dynamic "Write State.vi"("error in (no error)"=w2219, "State"=w2235, "State Machine in"=w2227) -> ("error out"=w2236:errorcluster, "State Machine out"=w2237:refnum<class "State Machine.lvclass">)  [unwired: 7 in]
            n1324 = call-dynamic "Write State Machine.vi"("error in (no error)"=w2236, "State Machine.lvclass"=w2237, "Device in"=w2238) -> ("error out"=w2233:errorcluster, "Device out"=w2234:refnum<class "Channel.lvclass">)  [unwired: 7 in]
          }
        }
        n1325 = call-dynamic "Write Channel.vi"("error in (no error)"=w1877, "Channel.lvclass"=w1878, "Acquisition in"=w2051) -> ("error out"=w2048:errorcluster, "Acquisition out"=w2047:refnum<class "Acquisition.lvclass">)  [unwired: 7 in]
        n1326 = call-dynamic "Write AcquisitionD.vi"("error in (no error)"=w2048, "Acquisition.lvclass"=w2047, "S4ACS_GUI in"=w2052) -> ("error out"=w2016:errorcluster, "S4ACS_GUI out"=w2020:refnum<class "S4GUI.lvclass">)  [unwired: 7 in]
        n1327 = Merge Errors(w2019, w2018, w2017, w2016) -> (w2015:errorcluster)
        n1328 = call "Write cfg file.vi"("error in (no error)"=w2015, "cfg file"="lastsaved.cfg", "S4ACS_GUI in"=w2020) -> ("error out"=w2102:errorcluster, "S4ACS_GUI out"=w2104:refnum<class "S4GUI.lvclass">)  [unwired: 7 in]
      }
      event "FTM", "AQM", "SZM", "EM Gain": Value Change {
        # "criar  S4GUI:CalcTemp.vi (metodo da classe S4GUI.lvclass)\na mesma lógica do Channel:ValidateConfig.vi usando\no cluster S4GUI:Parameters CCD em vez do cluster Interface:CCD CF.\nIgnore o Texp Min e apenas salve a temperatura em S4GUI:PrevTemp"
        # "Sinaliza que não há requisição de SET CCD mode"
        n1329 = event-data() -> ()  [unwired: 1 in, 6 out]
        n1330 = call-dynamic "Write SET request.vi"("error in (no error)"=w2296, "SET request"=FALSE, "S4GUI in"=w2298) -> ("error out"=w2295:errorcluster, "S4GUI out"=w2297:refnum<class "S4GUI.lvclass">)  [unwired: 7 in]
        n1331 = local read "EM Gain"() -> (w2300:u16)
        n1332 = local read "AQM"() -> (w2310:T4)
        n1333 = local read "SZM"() -> (w2309:T3)
        n1334 = local read "FTM"() -> (w2311:enum16{"OFF", "ON"})
        n1335 = call-dynamic "Read CCD mode.vi"("error in (no error)"=w2295, "S4GUI in"=w2297) -> ("error out"=w2308:errorcluster, "CCD mode"=w2313:T29, "S4GUI out"=w2314:refnum<class "S4GUI.lvclass">)  [unwired: 7 in]
        n1336 = Bundle By Name(cluster=w2313, "FTM"=w2311, "AQM"=w2310, "SZM"=w2309, "EM gain"=w2300) -> (w2312:T29)
        n1337 = call-dynamic "Write CCD mode.vi"("error in (no error)"=w2308, "CCD mode"=w2312, "S4GUI in"=w2314) -> ("error out"=w2306:errorcluster, "S4GUI out"=w2307:refnum<class "S4GUI.lvclass">)  [unwired: 7 in]
        n1338 = call-dynamic "LoadCCDmode.vi"("error in (no error)"=w2306, "S4GUI in"=w2307) -> ("error out"=w2304:errorcluster, "S4GUI out"=w2305:refnum<class "S4GUI.lvclass">)  [unwired: 8 in]
        n1339 = call-dynamic "Read Parameters CCD modes.vi"("error in (no error)"=w2304, "S4GUI in"=w2305) -> ("error out"=w2301:errorcluster, "Parameters CCD modes"=w2299:T5, "S4GUI out"=w2303:refnum<class "S4GUI.lvclass">)  [unwired: 7 in]
        n1340 = call-dynamic "Read InfoCCDmode.vi"("error in (no error)"=w2301, "S4GUI in"=w2303) -> ("error out"=w2291:errorcluster, "InfoCCDmode"=w2302:T2, "S4GUI out"=w2292:refnum<class "S4GUI.lvclass">)  [unwired: 7 in]
        n1341 = local write "Parameters CCD modes"(w2299) -> ()
        n1342 = local write "InfoCCDmode"(w2302) -> ()
        n1343 = call-dynamic "CalcTemp.vi"("error in (no error)"=w2291, "S4GUI in"=w2292) -> ("error out"=w2290:errorcluster, "S4GUI out"=w2289:refnum<class "S4GUI.lvclass">)  [unwired: 8 in]
        n1344 = call-dynamic "Read Prev Temp.vi"("error in (no error)"=w2290, "S4GUI in"=w2289) -> ("Prev Temp"=→"Preview Temp.":dbl)  [unwired: 7 in, 2 out]
      }
      event "TCS mode": Value Change {
        # "2024-04-04: Não se usa mais o ID para configurar a comunicação..."
        # "simul"
        # "real"
        # "Inicializar nova comunicação, de acordo\n com valor de TCS mode\n\nServer.Write id (T=6 ou F=12)\nTCS.Init"
        # "Parar a comunciação atual\nServer.End"
        n1345 = event-data() -> ("NewVal"=w2317:bool)  [unwired: 1 in, 5 out]
        n1346 = call-dynamic "Read TCS.lvclass.vi"("error in (no error)"=w2327, "S4GUI in"=w2328) -> ("error out"=w2322:errorcluster, "TCS.lvclass"=w2325:refnum<class "TCS.lvclass">, "S4GUI out"=w2326:refnum<class "S4GUI.lvclass">)  [unwired: 7 in]
        n1347 = call-dynamic "End.vi"("error in (no error)"=w2322, "Server in"=w2325) -> ("error out"=w2321:errorcluster, "Server out"=w2324:refnum<class "TCS.lvclass">)  [unwired: 8 in]
        n1348 = Select(t=u32 6, s=w2317, f=u32 12) -> (s? t:f=w2331:u32)
        n1349 = call-dynamic "Write id.vi"("error in (no error)"=w2321, "id"=w2331, "Server in"=w2324) -> ("error out"=w2320:errorcluster, "Server out"=w2323:refnum<class "TCS.lvclass">)  [unwired: 7 in]
        n1350 = call-dynamic "Initialize.vi"("error in (no error)"=w2320, "TCS in"=w2323) -> ("error out"=w2318:errorcluster, "TCS out"=w2319:refnum<class "TCS.lvclass">)  [unwired: 8 in]
        n1351 = call-dynamic "Write TCS.lvclass.vi"("error in (no error)"=w2318, "TCS.lvclass"=w2319, "S4GUI in"=w2326) -> ("error out"=w2315:errorcluster, "S4GUI out"=w2316:refnum<class "S4GUI.lvclass">)  [unwired: 7 in]
      }
      event "enter password": Value Change {
        n1352 = event-data() -> ("NewVal"=w2332:bool)  [unwired: 1 in]
        n1353 = case shown="True" w2332 {
          tunnel: [w2338 w2340] -> w2336
          tunnel: [w2337 w2339] -> w2335
          tunnel: w2334 -> [w2338 w2353]
          tunnel: w2333 -> [w2337 w2352]
          frame False {
          }
          frame True {
            # "Verifica senha de configuração de CCD do Administrador"
            n1354 = Equal?(x="password", y="camerasetup") -> (x = y?=w2350:bool)
            n1355 = call-dynamic "Write mode Adm.vi"("error in (no error)"=w2352, "mode Adm"=w2350, "S4GUI in"=w2353) -> ("error out"=w2341:errorcluster, "S4GUI out"=w2342:refnum<class "S4GUI.lvclass">)  [unwired: 7 in]
            n1356 = call-dynamic "Read mode Adm.vi"("error in (no error)"=w2341, "S4GUI in"=w2342) -> ("error out"=w2348:errorcluster, "mode Adm"=w2345:bool, "S4GUI out"=w2347:refnum<class "S4GUI.lvclass">)  [unwired: 7 in]
            n1357 = Select(t="Eng/Camera tab: password OK clicked successful" ("User Event"), s=w2345, f="Eng/Camera tab: password OK clicked with wrong input" ("User Event")) -> (s? t:f=w2346:string)
            n1358 = call-dynamic "Write User Event.vi"("error in (no error)"=w2348, "User Event"=w2346, "S4GUI in"=w2347) -> ("error out"=w2339:errorcluster, "S4GUI out"=w2340:refnum<class "S4GUI.lvclass">)  [unwired: 7 in]
          }
        }
      }
      event "enter password 2": Value Change {
        # "Verificação de senha na aba \"CCD modes\""
        n1359 = event-data() -> ("NewVal"=w2354:bool)  [unwired: 1 in]
        n1360 = case shown="True" w2354 {
          tunnel: [w2360 w2370] -> w2358
          tunnel: [w2359 w2369] -> w2357
          tunnel: w2356 -> [w2360 w2375]
          tunnel: w2355 -> [w2359 w2374]
          frame False {
          }
          frame True {
            # "Verifica senha de configuração de CCD do Administrador"
            n1361 = Equal?(x="password 2", y="ccdmodessetup") -> (x = y?=w2372:bool)
            n1362 = call-dynamic "Write mode Adm.vi"("error in (no error)"=w2374, "mode Adm"=w2372, "S4GUI in"=w2375) -> ("error out"=w2367:errorcluster, "S4GUI out"=w2368:refnum<class "S4GUI.lvclass">)  [unwired: 7 in]
            n1363 = call-dynamic "Read mode Adm.vi"("error in (no error)"=w2367, "S4GUI in"=w2368) -> ("error out"=w2365:errorcluster, "mode Adm"=w2362:bool, "S4GUI out"=w2366:refnum<class "S4GUI.lvclass">)  [unwired: 7 in]
            n1364 = Select(t="CCD mode tab: password OK clicked successful" ("User Event"), s=w2362, f="CCD mode tab: password OK clicked with wrong input" ("User Event")) -> (s? t:f=w2363:string)
            n1365 = call-dynamic "Write User Event.vi"("error in (no error)"=w2365, "User Event"=w2363, "S4GUI in"=w2366) -> ("error out"=w2369:errorcluster, "S4GUI out"=w2370:refnum<class "S4GUI.lvclass">)  [unwired: 7 in]
          }
        }
      }
      event "Tab ObsEng": Value Change {
        n1366 = event-data() -> ("NewVal"=w2376:enum32{"Obs", "CCD modes", "Eng"})  [unwired: 1 in]
        n1367 = case shown="\"Eng\"" w2376 {
          tunnel: [w2382 w2526 w2535] -> w2380
          tunnel: [w2384 w2524 w2534] -> w2379
          tunnel: w2378 -> [w2413 w2533 w2535]
          tunnel: w2377 -> [w2412 w2532 w2534]
          frame "CCD modes" {
            # "Sinaliza que não há requisição de SET CCD mode"
            # "Entrou na aba \"CCD modes\", ajusta para modo usuário normal..."
            n1368 = call-dynamic "Write mode Adm.vi"("error in (no error)"=w2412, "mode Adm"=FALSE, "S4GUI in"=w2413) -> ("error out"=w2407:errorcluster, "S4GUI out"=w2409:refnum<class "S4GUI.lvclass">)  [unwired: 7 in]
            n1369 = local write "password 2"("" ("password")) -> ()
            n1370 = call-dynamic "Write SET request.vi"("error in (no error)"=w2407, "SET request"=FALSE, "S4GUI in"=w2409) -> ("error out"=w2406:errorcluster, "S4GUI out"=w2408:refnum<class "S4GUI.lvclass">)  [unwired: 7 in]
            n1371 = disable-structure shown="Disabled" {
              frame Disabled {
                n1372 = flat-sequence {
                  tunnel: _ -> [w2420]
                  tunnel: [w2420] -> _
                  frame #0 {
                    n1373 = local read "AQM"() -> (w2417:T4)
                    n1374 = Less Or Equal?(x=w2417, y=T4."NORMAL FAINT: Conventional; 1 MHz; Gain 2") -> (x <= y?=w2416:bool)
                    n1375 = Select(t=w2417, s=w2416, f=T4."SLOW BRIGHT: Conventional; 0.1 MHz; Gain 1" ("y")) -> (s? t:f=w2418:T4)
                    n1376 = local write "EM Gain"(u16 2 ("EM Gain")) -> ()
                    n1377 = local write "AQM"(w2418) -> ()
                  }
                }
              }
              frame Enabled {
              }
            }
            n1378 = flat-sequence {
              tunnel: w2406 -> [w2423]
              tunnel: [w2423] -> w2391
              tunnel: [w2422] -> w2388
              tunnel: [w2421] -> w2389
              frame #0 {
                w2421 = u16 2 ("EM Gain")
                w2422 = T4."NORMAL FAINT: Conventional; 1 MHz; Gain 2" ("AQM")
                n1379 = local write "EM Gain"(w2421) -> ()
                n1380 = local write "AQM"(w2422) -> ()
              }
            }
            n1381 = call-dynamic "Read CCD mode.vi"("error in (no error)"=w2391, "S4GUI in"=w2408) -> ("error out"=w2397:errorcluster, "CCD mode"=w2394:T29, "S4GUI out"=w2393:refnum<class "S4GUI.lvclass">)  [unwired: 7 in]
            n1382 = local read "SZM"() -> (w2390:T3)
            n1383 = local read "FTM"() -> (w2396:enum16{"OFF", "ON"})
            n1384 = Bundle By Name(cluster=w2394, "FTM"=w2396, "SZM"=w2390, "EM gain"=w2389, "AQM"=w2388) -> (w2395:T29)
            n1385 = call-dynamic "Write CCD mode.vi"("error in (no error)"=w2397, "CCD mode"=w2395, "S4GUI in"=w2393) -> ("error out"=w2399:errorcluster, "S4GUI out"=w2398:refnum<class "S4GUI.lvclass">)  [unwired: 7 in]
            n1386 = call-dynamic "LoadCCDmode.vi"("error in (no error)"=w2399, "S4GUI in"=w2398) -> ("error out"=w2401:errorcluster, "S4GUI out"=w2400:refnum<class "S4GUI.lvclass">)  [unwired: 8 in]
            n1387 = call-dynamic "Read Parameters CCD modes.vi"("error in (no error)"=w2401, "S4GUI in"=w2400) -> ("error out"=w2404:errorcluster, "Parameters CCD modes"=w2392:T5, "S4GUI out"=w2402:refnum<class "S4GUI.lvclass">)  [unwired: 7 in]
            n1388 = local write "Parameters CCD modes"(w2392) -> ()
